vi "Set Max Retries.vi"(8 "error in":errorcluster, 10 "Max Retries":u8=3, 11 "Transfer Beginner in":refnum<class "Transfer Beginner.lvclass">) -> (0 "error out":errorcluster, 3 "Transfer Beginner out":refnum<class "Transfer Beginner.lvclass">)   [LabVIEW 2020, in "CANopen.lvlib" / "Transfer Beginner.lvlib" / "Transfer Beginner.lvclass"]
uses:
  Transfer Beginner.lvclass
  Transfer Beginner.lvclass/Transfer Beginner.ctl
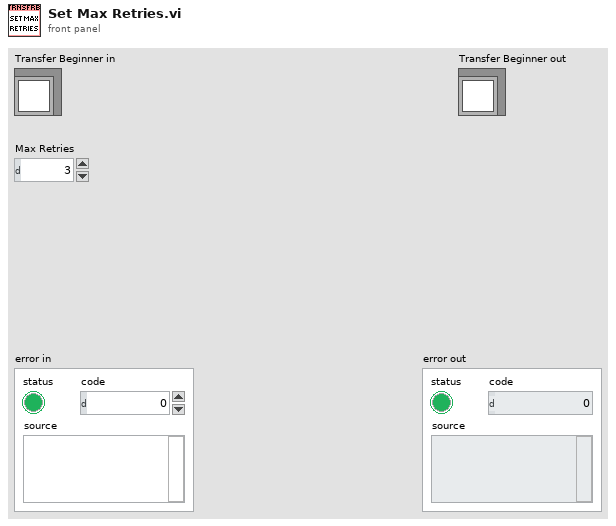
[diagram p1: front panel]
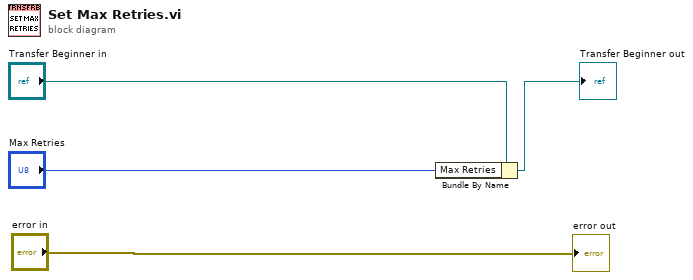
[diagram p0: block diagram]
diagram:
  n1 = Bundle By Name(cluster="Transfer Beginner in", "Max Retries"="Max Retries") -> (→"Transfer Beginner out":refnum<class "Transfer Beginner.lvclass">)
  "error out" <- "error in"
